vi "ListBox-Right click select.vi"(8 "error in":errorcluster, 9 "Coords":T1, 11 "ListBox ref":refnum<vi>) -> (0 "error out":errorcluster, 3 "ListBox ref":refnum<vi>)   [LabVIEW 2020]
uses:
  <vilib>/Utility/miscctls.llb/LVPoint32TypeDef.ctl
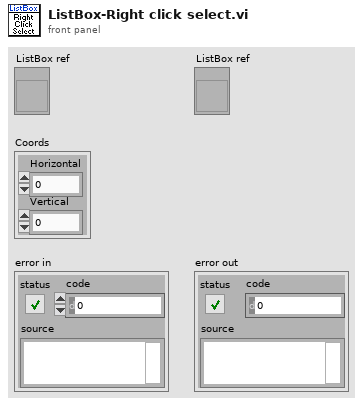
[diagram p1: front panel]
types:
  T1 = typedef "LVPoint32TypeDef.ctl" = cluster{"Horizontal":i32, "Vertical":i32}
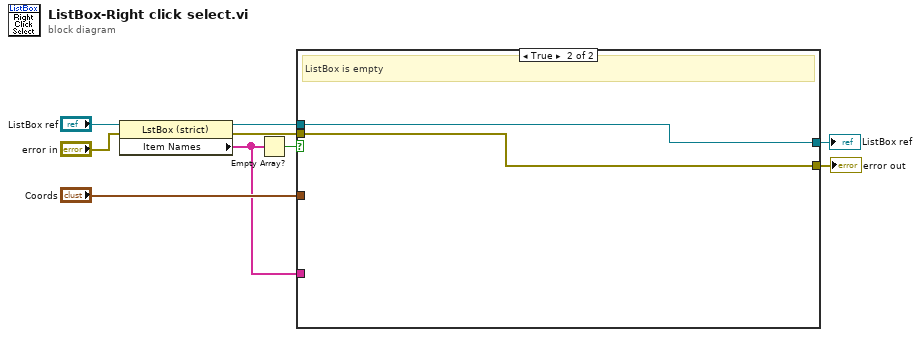
[diagram p0: block diagram]
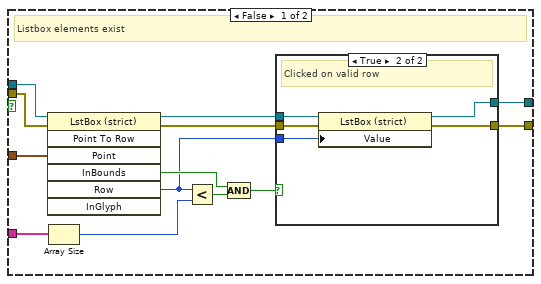
[diagram p2: hidden frame]
diagram:
  n1 = property on="Property Node" class="LstBox (strict)"(reference="ListBox ref", error in="error in") -> (reference out=w6:refnum<vi>, error out=w3:errorcluster, "Item Names"=w5:string[])
  n2 = Empty Array?(array=w5) -> (empty?=w4:bool)
  n3 = case shown="True" w4 {
    tunnel: "Coords" -> [w22 _]
    tunnel: [w18 w31] -> w8
    tunnel: w6 -> [w14 w30]
    tunnel: w5 -> [w12 _]
    tunnel: w3 -> [w11 w31]
    tunnel: [w10 w30] -> w1
    frame False {
      # "Listbox elements exist"
      n4 = invoke on="Invoke Node" class="LstBox (strict)" method="Point To Row"(reference=w14, error in=w11, "Point"=w22) -> (reference out=w17:refnum<vi>, error out=w19:errorcluster, "InBounds"=w20:bool, "Row"=w15:i32)  [unwired: 4 in, 3 out]
      n5 = Array Size(array=w12) -> (size(s)=w13:i32)
      n6 = Less?(x=w15, y=w13) -> (x < y?=w21:bool)
      n7 = Compound Arithmetic op=AND(w20, w21) -> (w16:bool)
      n8 = case shown="True" w16 {
        tunnel: w19 -> [w24 w29]
        tunnel: [w24 w28] -> w18
        tunnel: w17 -> [w23 w27]
        tunnel: w15 -> [_ w26]
        tunnel: [w23 w25] -> w10
        frame False {
          # "Invalid click"
        }
        frame True {
          # "Clicked on valid row"
          n9 = property class="LstBox (strict)"(reference=w27, error in=w29, "Value"=w26) -> (reference out=w25:refnum<vi>, error out=w28:errorcluster)
        }
      }
    }
    frame True {
      # "ListBox is empty"
    }
  }
  "error out" <- w8
  "ListBox ref" <- w1
